vi "Memory.Array.Subset.vi"(7 "length (-1: rest)":i64 format="%d bytes", 8 "error in (no error)":errorcluster, 9 "index (0)":u64, 11 "Array in":refnum<class "Memory.Array.lvclass">) -> (0 "error out":errorcluster, 2 "subset Array":refnum<class "Memory.Array.lvclass">, 3 "Array out":refnum<class "Memory.Array.lvclass">)   [LabVIEW 2016, in "LabVIEW Memory Manager.lvlib" / "Memory.Array.lvclass"]
uses:
  Memory.Array.lvclass
  Pointer/Memory.Pointer.Void.lvclass
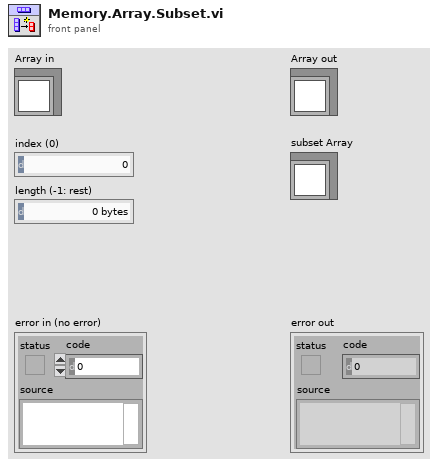
[diagram p1: front panel]
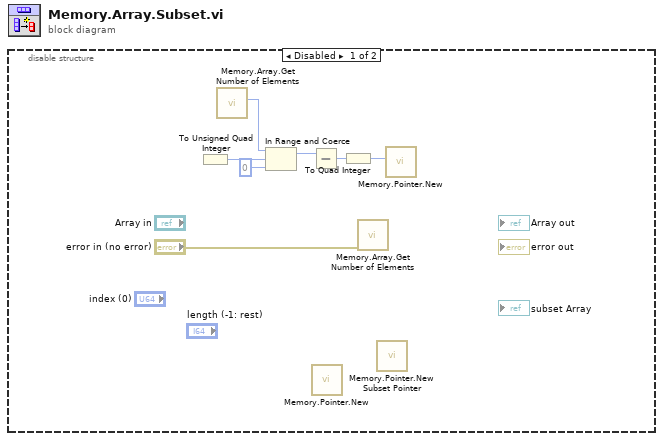
[diagram p0: block diagram]
diagram:
  n1 = disable-structure shown="Disabled" {
    frame Disabled {
      n2 = To Unsigned Quad Integer() -> (0:w6:u64)  [unwired: 1 in]
      n3 = call "Memory.Array.Get Number of Elements.vi"() -> ("number of elements"=w5:u64, "error in (no error)"=w9:errorcluster, "Memory.Array in"=w8:refnum<class "Memory.Array.lvclass">)  [unwired: 7 in, 2 out]
      n4 = In Range and Coerce(upper limit=w5, x=w6, lower limit=u64 0) -> (coerced(x)=w3:u64)  [unwired: 1 out]
      n5 = Subtract(x=w3) -> (y=w7:u64, x-y=w2:u64)
      n6 = call "Memory.Pointer.New.vi"() -> ()  [unwired: 9 in, 3 out]
      n7 = To Quad Integer(1:w2) -> (0:w1:i64)
      n8 = call "Memory.Array.Get Number of Elements.vi"("error in (no error)"="error in (no error)") -> ()  [unwired: 8 in, 3 out]
      n9 = call "Memory.Pointer.New Subset Pointer.vi"() -> ()  [unwired: 9 in, 3 out]
      n10 = call "Memory.Pointer.New.vi"("size"=w1) -> ()  [unwired: 8 in, 3 out]
    }
    frame Enabled {
    }
  }
